vi "RUN.vi"(8 "error in (no error)":errorcluster, 11 "Interface in":refnum<class "Interface.lvclass">) -> (0 "error out":errorcluster, 3 "Interface out":refnum<class "Interface.lvclass">)   [LabVIEW 2018, in "Interface.lvclass"]
uses:
  Interface.lvclass
  Interface.lvclass/Interface.ctl
  State Machine/State Machine.lvclass/State Machine.ctl
  CCD/CCD.lvclass/CCD.ctl
  State Machine/State Machine.lvclass
  CCD/CCD.lvclass
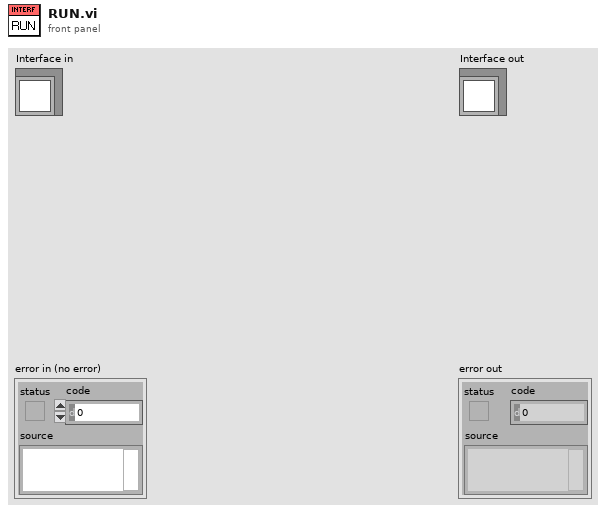
[diagram p1: front panel]
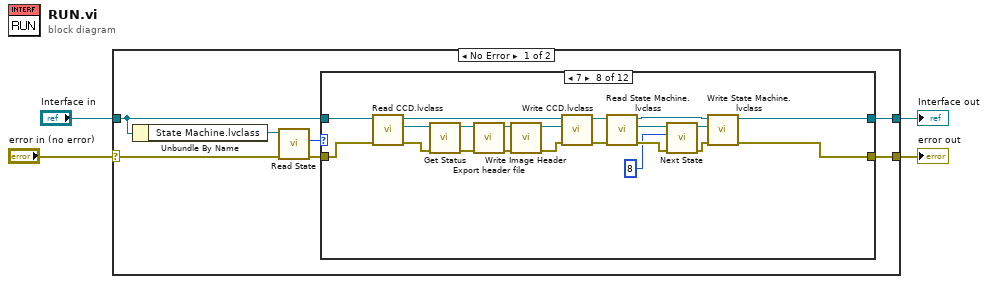
[diagram p0: block diagram]
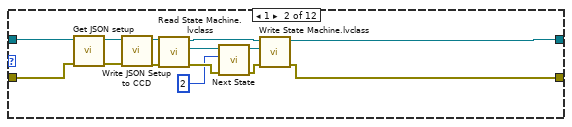
[diagram p3: hidden frame]
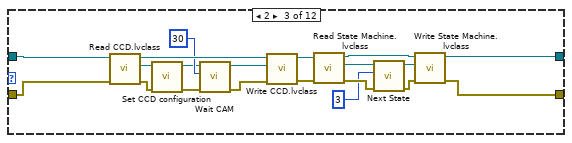
[diagram p4: hidden frame]
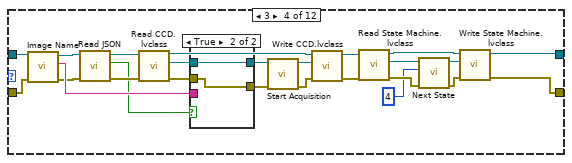
[diagram p5: hidden frame]
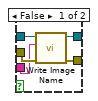
[diagram p6: hidden frame]
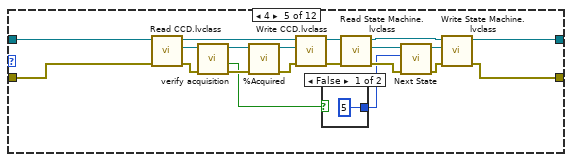
[diagram p7: hidden frame]
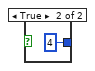
[diagram p8: hidden frame]
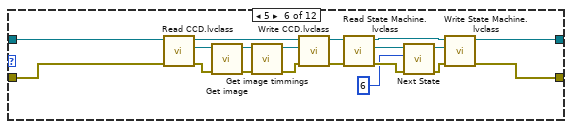
[diagram p9: hidden frame]
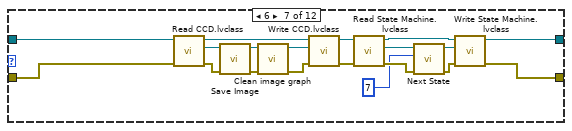
[diagram p10: hidden frame]
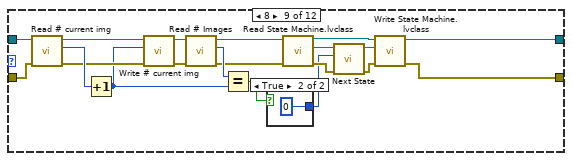
[diagram p11: hidden frame]
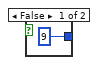
[diagram p12: hidden frame]
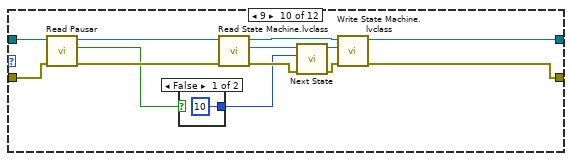
[diagram p13: hidden frame]
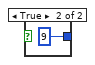
[diagram p14: hidden frame]
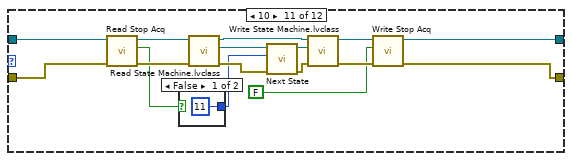
[diagram p15: hidden frame]
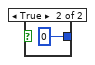
[diagram p16: hidden frame]
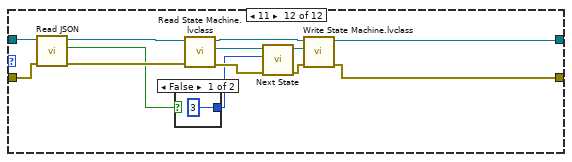
[diagram p17: hidden frame]
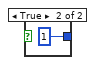
[diagram p18: hidden frame]
diagram:
  n1 = case shown="No Error" "error in (no error)" {
    selector: "error in (no error)" -> [w10 w232]
    tunnel: [w5 w232] -> w3
    tunnel: [w6 w231] -> w1
    tunnel: "Interface in" -> [w8 w231]
    frame No Error {
      n2 = Unbundle By Name(w8) -> ("State Machine.lvclass"=w11:refnum<class "State Machine.lvclass">)
      n3 = call "Read State.vi"("error in (no error)"=w10, "State Machine in"=w11) -> ("error out"=w7:errorcluster, "State"=w9:u16)  [unwired: 7 in, 1 out]
      n4 = case shown="7" w9 {
        tunnel: w8 -> [w13 w15 w47 w59 w92 w105 w130 w151 w180 w195 w206 w220]
        tunnel: [w13 w19 w30 w61 w81 w103 w128 w149 w162 w185 w200 w222] -> w6
        tunnel: w7 -> [w12 w14 w45 w58 w91 w104 w129 w150 w179 w194 w207 w219]
        tunnel: [w12 w18 w29 w60 w80 w102 w127 w148 w161 w184 w199 w221] -> w5
        frame 0, Default {
        }
        frame 1 {
          n5 = call "Get JSON setup.vi"("error in (no error)"=w14, "Interface in"=w15) -> ("error out"=w17:errorcluster, "Interface out"=w16:refnum<class "Interface.lvclass">)  [unwired: 8 in]
          n6 = call "Write JSON Setup to CCD.vi"("error in (no error)"=w17, "Interface in"=w16) -> ("error out"=w20:errorcluster, "Interface out"=w21:refnum<class "Interface.lvclass">)  [unwired: 8 in]
          n7 = call "Read State Machine.lvclass.vi"("error in (no error)"=w20, "Interface in"=w21) -> ("error out"=w26:errorcluster, "State Machine.lvclass"=w23:refnum<class "State Machine.lvclass">, "Interface out"=w27:refnum<class "Interface.lvclass">)  [unwired: 7 in]
          n8 = call "Next State.vi"("error in (no error)"=w26, "New_State"=2, "State Machine in"=w23) -> ("error out"=w25:errorcluster, "State Machine out"=w24:refnum<class "State Machine.lvclass">)  [unwired: 7 in]
          n9 = call "Write State Machine.lvclass.vi"("error in (no error)"=w25, "State Machine.lvclass"=w24, "Interface in"=w27) -> ("error out"=w18:errorcluster, "Interface out"=w19:refnum<class "Interface.lvclass">)  [unwired: 7 in]
        }
        frame 2 {
          n10 = call "Read CCD.lvclass.vi"("error in (no error)"=w45, "Interface in"=w47) -> ("error out"=w39:errorcluster, "CCD.lvclass"=w28:refnum<class "CCD.lvclass">, "Interface out"=w46:refnum<class "Interface.lvclass">)  [unwired: 7 in]
          n11 = call "Set CCD configuration.vi"("error in (no error)"=w39, "CCD in"=w28) -> ("error out"=w40:errorcluster, "CCD out"=w43:refnum<class "CCD.lvclass">)  [unwired: 8 in]
          n12 = call "Wait CAM.vi"("error in (no error)"=w40, "Numeric Control"=u16 30, "CCD in"=w43) -> ("error out"=w41:errorcluster, "CCD out"=w42:refnum<class "CCD.lvclass">)  [unwired: 7 in]
          n13 = call "Write CCD.lvclass.vi"("error in (no error)"=w41, "CCD.lvclass"=w42, "Interface in"=w46) -> ("error out"=w32:errorcluster, "Interface out"=w31:refnum<class "Interface.lvclass">)  [unwired: 7 in]
          n14 = call "Read State Machine.lvclass.vi"("error in (no error)"=w32, "Interface in"=w31) -> ("error out"=w37:errorcluster, "State Machine.lvclass"=w34:refnum<class "State Machine.lvclass">, "Interface out"=w38:refnum<class "Interface.lvclass">)  [unwired: 7 in]
          n15 = call "Next State.vi"("error in (no error)"=w37, "New_State"=3, "State Machine in"=w34) -> ("error out"=w36:errorcluster, "State Machine out"=w35:refnum<class "State Machine.lvclass">)  [unwired: 7 in]
          n16 = call "Write State Machine.lvclass.vi"("error in (no error)"=w36, "State Machine.lvclass"=w35, "Interface in"=w38) -> ("error out"=w29:errorcluster, "Interface out"=w30:refnum<class "Interface.lvclass">)  [unwired: 7 in]
        }
        frame 3 {
          n17 = call "Image Name.vi"("error in (no error)"=w58, "Interface in"=w59) -> ("error out"=w50:errorcluster, "Image Name"=w53:string, "Interface out"=w52:refnum<class "Interface.lvclass">)  [unwired: 7 in]
          n18 = call "Read JSON.vi"("error in (no error)"=w50, "Interface in"=w52) -> ("error out"=w49:errorcluster, "JSON"=w48:bool, "Interface out"=w51:refnum<class "Interface.lvclass">)  [unwired: 7 in]
          n19 = call "Read CCD.lvclass.vi"("error in (no error)"=w49, "Interface in"=w51) -> ("error out"=w55:errorcluster, "CCD.lvclass"=w54:refnum<class "CCD.lvclass">, "Interface out"=w72:refnum<class "Interface.lvclass">)  [unwired: 7 in]
          n20 = case shown="True" w48 {
            tunnel: [w77 w79] -> w57
            tunnel: [w76 w78] -> w56
            tunnel: w55 -> [w75 w79]
            tunnel: w54 -> [w74 w78]
            tunnel: w53 -> [w73 _]
            frame False {
              n21 = call "Write Image Name.vi"("error in (no error)"=w75, "Image Name"=w73, "CCD in"=w74) -> ("error out"=w77:errorcluster, "CCD out"=w76:refnum<class "CCD.lvclass">)  [unwired: 7 in]
            }
            frame True {
            }
          }
          n22 = call "Start Acquisition.vi"("error in (no error)"=w57, "CCD in"=w56) -> ("error out"=w71:errorcluster, "CCD out"=w70:refnum<class "CCD.lvclass">)  [unwired: 8 in]
          n23 = call "Write CCD.lvclass.vi"("error in (no error)"=w71, "CCD.lvclass"=w70, "Interface in"=w72) -> ("error out"=w63:errorcluster, "Interface out"=w62:refnum<class "Interface.lvclass">)  [unwired: 7 in]
          n24 = call "Read State Machine.lvclass.vi"("error in (no error)"=w63, "Interface in"=w62) -> ("error out"=w68:errorcluster, "State Machine.lvclass"=w65:refnum<class "State Machine.lvclass">, "Interface out"=w69:refnum<class "Interface.lvclass">)  [unwired: 7 in]
          n25 = call "Next State.vi"("error in (no error)"=w68, "New_State"=4, "State Machine in"=w65) -> ("error out"=w67:errorcluster, "State Machine out"=w66:refnum<class "State Machine.lvclass">)  [unwired: 7 in]
          n26 = call "Write State Machine.lvclass.vi"("error in (no error)"=w67, "State Machine.lvclass"=w66, "Interface in"=w69) -> ("error out"=w60:errorcluster, "Interface out"=w61:refnum<class "Interface.lvclass">)  [unwired: 7 in]
        }
        frame 4 {
          n27 = call "Read CCD.lvclass.vi"("error in (no error)"=w91, "Interface in"=w92) -> ("error out"=w95:errorcluster, "CCD.lvclass"=w94:refnum<class "CCD.lvclass">, "Interface out"=w93:refnum<class "Interface.lvclass">)  [unwired: 7 in]
          n28 = call "verify acquisition"("error in (no error)"=w95, "CCD in"=w94) -> ("error out"=w97:errorcluster, "Acquiring"=w83:bool, "CCD out"=w96:refnum<class "CCD.lvclass">)  [unwired: 7 in]
          n29 = call "%Acquired.vi"("error in (no error)"=w97, "CCD in"=w96) -> ("error out"=w99:errorcluster, "CCD out"=w98:refnum<class "CCD.lvclass">)  [unwired: 8 in]
          n30 = call "Write CCD.lvclass.vi"("error in (no error)"=w99, "CCD.lvclass"=w98, "Interface in"=w93) -> ("error out"=w90:errorcluster, "Interface out"=w89:refnum<class "Interface.lvclass">)  [unwired: 7 in]
          n31 = case shown="False" w83 {
            tunnel: [5 4] -> w82
            frame False {
            }
            frame True {
            }
          }
          n32 = call "Read State Machine.lvclass.vi"("error in (no error)"=w90, "Interface in"=w89) -> ("error out"=w85:errorcluster, "State Machine.lvclass"=w88:refnum<class "State Machine.lvclass">, "Interface out"=w84:refnum<class "Interface.lvclass">)  [unwired: 7 in]
          n33 = call "Next State.vi"("error in (no error)"=w85, "New_State"=w82, "State Machine in"=w88) -> ("error out"=w86:errorcluster, "State Machine out"=w87:refnum<class "State Machine.lvclass">)  [unwired: 7 in]
          n34 = call "Write State Machine.lvclass.vi"("error in (no error)"=w86, "State Machine.lvclass"=w87, "Interface in"=w84) -> ("error out"=w80:errorcluster, "Interface out"=w81:refnum<class "Interface.lvclass">)  [unwired: 7 in]
        }
        frame 5 {
          n35 = call "Read CCD.lvclass.vi"("error in (no error)"=w104, "Interface in"=w105) -> ("error out"=w116:errorcluster, "CCD.lvclass"=w115:refnum<class "CCD.lvclass">, "Interface out"=w114:refnum<class "Interface.lvclass">)  [unwired: 7 in]
          n36 = call "Get image.vi"("error in (no error)"=w116, "CCD in"=w115) -> ("error out"=w117:errorcluster, "CCD out"=w118:refnum<class "CCD.lvclass">)  [unwired: 8 in]
          n37 = call "Get image timmings.vi"("error in (no error)"=w117, "CCD in"=w118) -> ("error out"=w120:errorcluster, "CCD out"=w119:refnum<class "CCD.lvclass">)  [unwired: 8 in]
          n38 = call "Write CCD.lvclass.vi"("error in (no error)"=w120, "CCD.lvclass"=w119, "Interface in"=w114) -> ("error out"=w113:errorcluster, "Interface out"=w112:refnum<class "Interface.lvclass">)  [unwired: 7 in]
          n39 = call "Read State Machine.lvclass.vi"("error in (no error)"=w113, "Interface in"=w112) -> ("error out"=w108:errorcluster, "State Machine.lvclass"=w111:refnum<class "State Machine.lvclass">, "Interface out"=w107:refnum<class "Interface.lvclass">)  [unwired: 7 in]
          n40 = call "Next State.vi"("error in (no error)"=w108, "New_State"=6, "State Machine in"=w111) -> ("error out"=w109:errorcluster, "State Machine out"=w110:refnum<class "State Machine.lvclass">)  [unwired: 7 in]
          n41 = call "Write State Machine.lvclass.vi"("error in (no error)"=w109, "State Machine.lvclass"=w110, "Interface in"=w107) -> ("error out"=w102:errorcluster, "Interface out"=w103:refnum<class "Interface.lvclass">)  [unwired: 7 in]
        }
        frame 6 {
          n42 = call "Read CCD.lvclass.vi"("error in (no error)"=w129, "Interface in"=w130) -> ("error out"=w125:errorcluster, "CCD.lvclass"=w126:refnum<class "CCD.lvclass">, "Interface out"=w139:refnum<class "Interface.lvclass">)  [unwired: 7 in]
          n43 = call "Save Image.vi"("error in (no error)"=w125, "CCD in"=w126) -> ("error out"=w121:errorcluster, "CCD out"=w124:refnum<class "CCD.lvclass">)  [unwired: 8 in]
          n44 = call "Clean image graph.vi"("error in (no error)"=w121, "CCD in"=w124) -> ("error out"=w122:errorcluster, "CCD out"=w123:refnum<class "CCD.lvclass">)  [unwired: 8 in]
          n45 = call "Write CCD.lvclass.vi"("error in (no error)"=w122, "CCD.lvclass"=w123, "Interface in"=w139) -> ("error out"=w138:errorcluster, "Interface out"=w137:refnum<class "Interface.lvclass">)  [unwired: 7 in]
          n46 = call "Read State Machine.lvclass.vi"("error in (no error)"=w138, "Interface in"=w137) -> ("error out"=w133:errorcluster, "State Machine.lvclass"=w136:refnum<class "State Machine.lvclass">, "Interface out"=w132:refnum<class "Interface.lvclass">)  [unwired: 7 in]
          n47 = call "Next State.vi"("error in (no error)"=w133, "New_State"=7, "State Machine in"=w136) -> ("error out"=w134:errorcluster, "State Machine out"=w135:refnum<class "State Machine.lvclass">)  [unwired: 7 in]
          n48 = call "Write State Machine.lvclass.vi"("error in (no error)"=w134, "State Machine.lvclass"=w135, "Interface in"=w132) -> ("error out"=w127:errorcluster, "Interface out"=w128:refnum<class "Interface.lvclass">)  [unwired: 7 in]
        }
        frame 7 {
          n49 = call "Read CCD.lvclass.vi"("error in (no error)"=w150, "Interface in"=w151) -> ("error out"=w140:errorcluster, "CCD.lvclass"=w143:refnum<class "CCD.lvclass">, "Interface out"=w160:refnum<class "Interface.lvclass">)  [unwired: 7 in]
          n50 = call "Get Status.vi"("error in (no error)"=w140, "CCD in"=w143) -> ("error out"=w141:errorcluster, "CCD out"=w142:refnum<class "CCD.lvclass">)  [unwired: 7 in, 1 out]
          n51 = call "Export header file.vi"("error in (no error)"=w141, "CCD in"=w142) -> ("error out"=w147:errorcluster, "CCD out"=w146:refnum<class "CCD.lvclass">)  [unwired: 8 in]
          n52 = call "Write Image Header.vi"("error in (no error)"=w147, "CCD in"=w146) -> ("error out"=w144:errorcluster, "CCD out"=w145:refnum<class "CCD.lvclass">)  [unwired: 8 in]
          n53 = call "Write CCD.lvclass.vi"("error in (no error)"=w144, "CCD.lvclass"=w145, "Interface in"=w160) -> ("error out"=w159:errorcluster, "Interface out"=w158:refnum<class "Interface.lvclass">)  [unwired: 7 in]
          n54 = call "Read State Machine.lvclass.vi"("error in (no error)"=w159, "Interface in"=w158) -> ("error out"=w154:errorcluster, "State Machine.lvclass"=w157:refnum<class "State Machine.lvclass">, "Interface out"=w153:refnum<class "Interface.lvclass">)  [unwired: 7 in]
          n55 = call "Next State.vi"("error in (no error)"=w154, "New_State"=8, "State Machine in"=w157) -> ("error out"=w155:errorcluster, "State Machine out"=w156:refnum<class "State Machine.lvclass">)  [unwired: 7 in]
          n56 = call "Write State Machine.lvclass.vi"("error in (no error)"=w155, "State Machine.lvclass"=w156, "Interface in"=w153) -> ("error out"=w148:errorcluster, "Interface out"=w149:refnum<class "Interface.lvclass">)  [unwired: 7 in]
        }
        frame 8 {
          n57 = call "Read # current img.vi"("error in (no error)"=w179, "Interface in"=w180) -> ("error out"=w176:errorcluster, "# current img"=w178:u16, "Interface out"=w177:refnum<class "Interface.lvclass">)  [unwired: 7 in]
          n58 = Increment(x=w178) -> (x+1=w171:u16)
          n59 = call "Write # current img.vi"("error in (no error)"=w176, "# current img"=w171, "Interface in"=w177) -> ("error out"=w175:errorcluster, "Interface out"=w174:refnum<class "Interface.lvclass">)  [unwired: 7 in]
          n60 = call "Read # Images.vi"("error in (no error)"=w175, "Interface in"=w174) -> ("error out"=w164:errorcluster, "# Images"=w172:u16, "Interface out"=w165:refnum<class "Interface.lvclass">)  [unwired: 7 in]
          n61 = Equal?(x=w172, y=w171) -> (x = y?=w173:bool)
          n62 = case shown="True" w173 {
            tunnel: [9 0] -> w163
            frame False {
            }
            frame True {
            }
          }
          n63 = call "Read State Machine.lvclass.vi"("error in (no error)"=w164, "Interface in"=w165) -> ("error out"=w167:errorcluster, "State Machine.lvclass"=w170:refnum<class "State Machine.lvclass">, "Interface out"=w166:refnum<class "Interface.lvclass">)  [unwired: 7 in]
          n64 = call "Next State.vi"("error in (no error)"=w167, "New_State"=w163, "State Machine in"=w170) -> ("error out"=w168:errorcluster, "State Machine out"=w169:refnum<class "State Machine.lvclass">)  [unwired: 7 in]
          n65 = call "Write State Machine.lvclass.vi"("error in (no error)"=w168, "State Machine.lvclass"=w169, "Interface in"=w166) -> ("error out"=w161:errorcluster, "Interface out"=w162:refnum<class "Interface.lvclass">)  [unwired: 7 in]
        }
        frame 9 {
          n66 = call "Read Pausar.vi"("error in (no error)"=w194, "Interface in"=w195) -> ("error out"=w187:errorcluster, "Pausar"=w183:bool, "Interface out"=w186:refnum<class "Interface.lvclass">)  [unwired: 7 in]
          n67 = case shown="False" w183 {
            tunnel: [10 9] -> w188
            frame False {
            }
            frame True {
            }
          }
          n68 = call "Read State Machine.lvclass.vi"("error in (no error)"=w187, "Interface in"=w186) -> ("error out"=w190:errorcluster, "State Machine.lvclass"=w193:refnum<class "State Machine.lvclass">, "Interface out"=w189:refnum<class "Interface.lvclass">)  [unwired: 7 in]
          n69 = call "Next State.vi"("error in (no error)"=w190, "New_State"=w188, "State Machine in"=w193) -> ("error out"=w191:errorcluster, "State Machine out"=w192:refnum<class "State Machine.lvclass">)  [unwired: 7 in]
          n70 = call "Write State Machine.lvclass.vi"("error in (no error)"=w191, "State Machine.lvclass"=w192, "Interface in"=w189) -> ("error out"=w184:errorcluster, "Interface out"=w185:refnum<class "Interface.lvclass">)  [unwired: 7 in]
        }
        frame 10 {
          n71 = call "Read Stop Acq.vi"("error in (no error)"=w207, "Interface in"=w206) -> ("error out"=w204:errorcluster, "Stop Acq"=w203:bool, "Interface out"=w205:refnum<class "Interface.lvclass">)  [unwired: 7 in]
          n72 = case shown="False" w203 {
            tunnel: [11 0] -> w208
            frame False {
            }
            frame True {
            }
          }
          n73 = call "Read State Machine.lvclass.vi"("error in (no error)"=w204, "Interface in"=w205) -> ("error out"=w210:errorcluster, "State Machine.lvclass"=w213:refnum<class "State Machine.lvclass">, "Interface out"=w209:refnum<class "Interface.lvclass">)  [unwired: 7 in]
          n74 = call "Next State.vi"("error in (no error)"=w210, "New_State"=w208, "State Machine in"=w213) -> ("error out"=w211:errorcluster, "State Machine out"=w212:refnum<class "State Machine.lvclass">)  [unwired: 7 in]
          n75 = call "Write State Machine.lvclass.vi"("error in (no error)"=w211, "State Machine.lvclass"=w212, "Interface in"=w209) -> ("error out"=w201:errorcluster, "Interface out"=w202:refnum<class "Interface.lvclass">)  [unwired: 7 in]
          n76 = call "Write Stop Acq.vi"("error in (no error)"=w201, "Stop Acq"=FALSE, "Interface in"=w202) -> ("error out"=w199:errorcluster, "Interface out"=w200:refnum<class "Interface.lvclass">)  [unwired: 7 in]
        }
        frame 11 {
          n77 = call "Read JSON.vi"("error in (no error)"=w219, "Interface in"=w220) -> ("error out"=w218:errorcluster, "JSON"=w216:bool, "Interface out"=w217:refnum<class "Interface.lvclass">)  [unwired: 7 in]
          n78 = case shown="False" w216 {
            tunnel: [3 1] -> w223
            frame False {
            }
            frame True {
            }
          }
          n79 = call "Read State Machine.lvclass.vi"("error in (no error)"=w218, "Interface in"=w217) -> ("error out"=w225:errorcluster, "State Machine.lvclass"=w228:refnum<class "State Machine.lvclass">, "Interface out"=w224:refnum<class "Interface.lvclass">)  [unwired: 7 in]
          n80 = call "Next State.vi"("error in (no error)"=w225, "New_State"=w223, "State Machine in"=w228) -> ("error out"=w226:errorcluster, "State Machine out"=w227:refnum<class "State Machine.lvclass">)  [unwired: 7 in]
          n81 = call "Write State Machine.lvclass.vi"("error in (no error)"=w226, "State Machine.lvclass"=w227, "Interface in"=w224) -> ("error out"=w221:errorcluster, "Interface out"=w222:refnum<class "Interface.lvclass">)  [unwired: 7 in]
        }
      }
    }
    frame Error {
    }
  }
  "error out" <- w3
  "Interface out" <- w1
